vi "CalculateMeasurementTimePre.vi"(2 "error out 2":errorcluster) -> (0 "error out":errorcluster)   [LabVIEW 2011]
uses:
  Variables/GlobalSetGetConfigureCamera.vi
  Variables/GlobalSetGetPixelOfRoi.vi
  Variables/GlobalGetSetMeasurementTimings.vi
  Variables/GetCalculateScanningParameter.vi
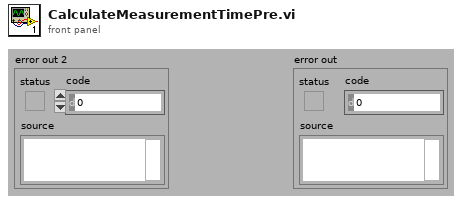
[diagram p1: front panel]
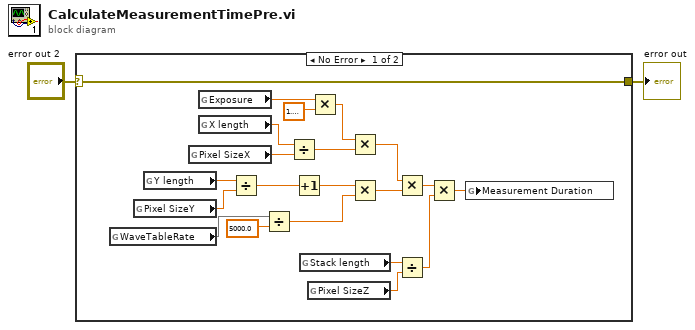
[diagram p0: block diagram]
diagram:
  n1 = case shown="No Error" "error out 2" {
    selector: "error out 2" -> [w21 w24]
    tunnel: [w21 w24] -> w1
    frame No Error {
      n2 = global read "GetCalculateScanningParameter.vi" "WaveTableRate"() -> (w6)
      n3 = global read "GlobalSetGetPixelOfRoi.vi" "Pixel SizeY"() -> (w10:dbl)
      n4 = global read "GlobalSetGetPixelOfRoi.vi" "Y length"() -> (w12:dbl)
      n5 = global read "GlobalSetGetPixelOfRoi.vi" "Pixel SizeX"() -> (w11:dbl)
      n6 = global read "GlobalSetGetConfigureCamera.vi" "Exposure"() -> (w22:sgl)
      n7 = global read "GlobalSetGetPixelOfRoi.vi" "X length"() -> (w13:dbl)
      n8 = Divide(x=w12, y=w10) -> (x/y=w15:dbl)
      n9 = Divide(x=w6, y=5000.0 ("x")) -> (x/y=w7:dbl)
      n10 = Divide(x=w13, y=w11) -> (x/y=w16:dbl)
      n11 = Increment(x=w15) -> (x+1=w18:dbl)
      n12 = global read "GlobalSetGetPixelOfRoi.vi" "Stack length"() -> (w9:dbl)
      n13 = global read "GlobalSetGetPixelOfRoi.vi" "Pixel SizeZ"() -> (w8:dbl)
      n14 = Multiply(x=w22, y=sgl 1.2) -> (x*y=w4:sgl)
      n15 = Multiply(x=w4, y=w16) -> (x*y=w20:dbl)
      n16 = Multiply(x=w18, y=w7) -> (x*y=w19:dbl)
      n17 = Multiply(x=w20, y=w19) -> (x*y=w17:dbl)
      n18 = Divide(x=w9, y=w8) -> (x/y=w14:dbl)
      n19 = Multiply(x=w17, y=w14) -> (x*y=w3:dbl)
      n20 = global write "GlobalGetSetMeasurementTimings.vi" "Measurement Duration"(w3) -> ()
    }
    frame Error {
    }
  }
  "error out" <- w1
